vi "Associate Instruments to Paths.vi"(0 "SA Path Group in":refnum<class "SA Path Group.lvclass">, 5 "TSM Context":T1, 11 "error in":errorcluster) -> (4 "SA Path Group out":refnum<class "SA Path Group.lvclass">, 15 "error out":errorcluster)   [LabVIEW 2023, in "RFFixtureCharact.PXI.lvlib" / "SA Path Group.lvclass"]
uses:
  SA Path Group.lvclass
  SA Path Group.lvclass/SA Path Group.ctl
  Public/Base Classes/Scalar/SA Path/SA Path.lvclass
  <vilib>/NI_TestStand_SemiconductorModule/NI_TestStand_Semiconductor_Module.lvlibp
  Common/Base Classes/Path Group/Path Group.lvclass
  <vilib>/addons/_RFCalAndCharactDatabase/NI_RFCalAndCharact_Database_API.lvlibp/Characterization/Characterization.lvlib
  Common/RFCalAndFixtureCharact.Common.lvlib
  <vilib>/NI_TestStand_SemiconductorModule/NI_TestStand_Semiconductor_Module.lvlibp/PinMap/RF/RFmx/PinToNIRFmxSession.vi
  <vilib>/NI_TestStand_SemiconductorModule/NI_TestStand_Semiconductor_Module.lvlibp/PinMap/RF/RFSG/PinToNIRFSGSession.vi
  Public/Charact Result Accessor/Scalar/Scalar Charact Result Accessor.lvclass
  C:/rfcal/AuxTools/STSRFFixtureCharactUtility/Source/Code Modules/Fixture/Public/Charact Result Accessor/Base/Charact Result Accessor.lvclass
  C:/rfcal/AuxTools/STSRFFixtureCharactUtility/Source/Code Modules/Common/Result Accessor/Result Accessor.lvclass
  C:/rfcal/AuxTools/STSRFFixtureCharactUtility/Source/Code Modules/Fixture/Public/Charact Result Accessor/Scalar/Scalar Charact Result Accessor.lvclass
  C:/rfcal/AuxTools/STSRFFixtureCharactUtility/Source/Code Modules/Fixture/Public/Base Classes/Scalar/SA Abstract Path/SA Abstract Path.lvclass
  C:/rfcal/AuxTools/STSRFFixtureCharactUtility/Source/Code Modules/Fixture/Public/Base Classes/Scalar/Scalar Path/Scalar Path.lvclass
  C:/rfcal/AuxTools/STSRFFixtureCharactUtility/Source/Code Modules/Common/Base Classes/Path/Path.lvclass
  C:/rfcal/AuxTools/STSRFFixtureCharactUtility/Source/Code Modules/Fixture/Public/Base Classes/Scalar/SA Path/SA Path.lvclass
  <vilib>/NI_TestStand_SemiconductorModule/NI_TestStand_Semiconductor_Module.lvlibp/PinMap/General/SemiconductorModuleContext.ctl
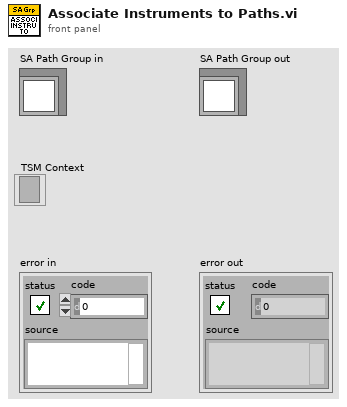
[diagram p1: front panel]
types:
  T1 = typedef "NI_TestStand_Semiconductor_Module.lvlibp/SemiconductorModuleContext.ctl" = refnum<k7>
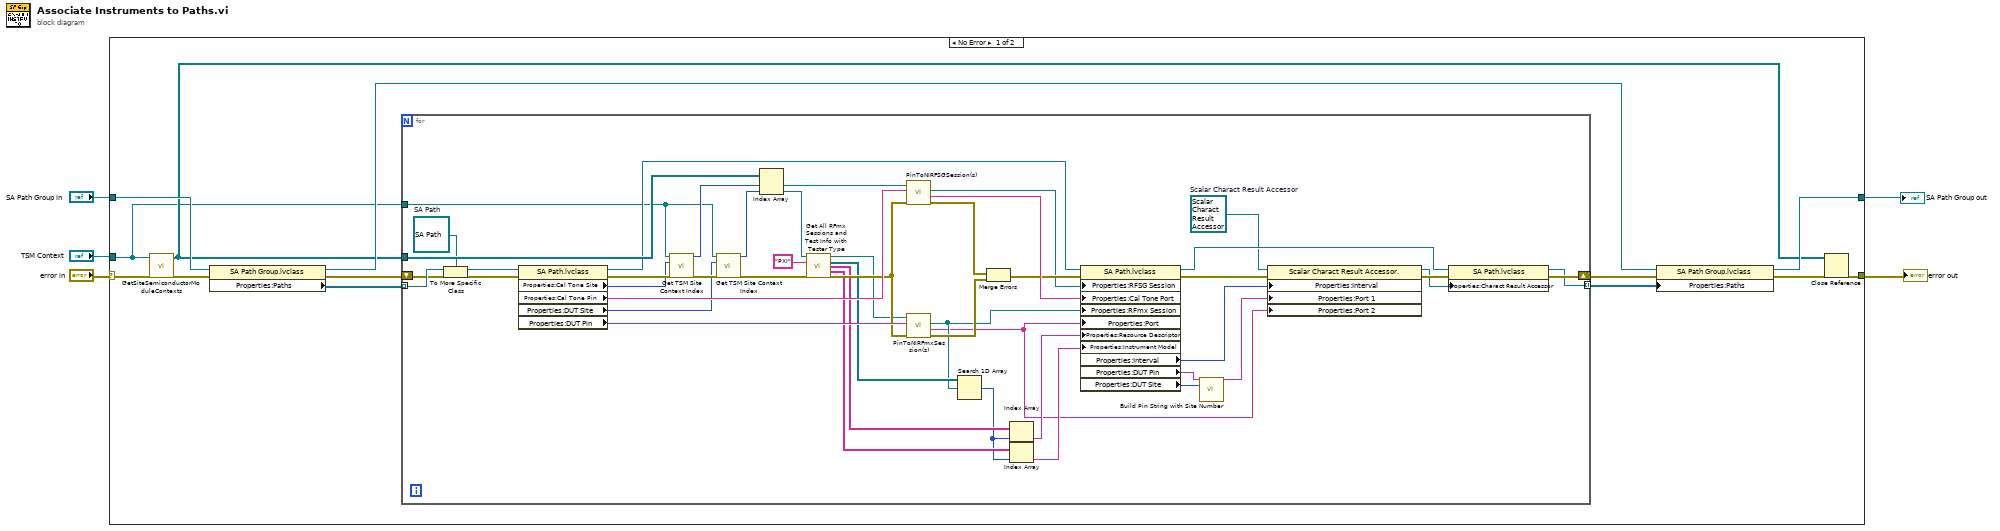
[diagram p0: block diagram]
diagram:
  n1 = case shown="No Error" "error in" {
    selector: "error in" -> [w10 w66]
    tunnel: "TSM Context" -> [w6 _]
    tunnel: "SA Path Group in" -> [w9 w65]
    tunnel: [w8 w66] -> w2
    tunnel: [w11 w65] -> w1
    frame No Error {
      n2 = call <vilib>:"GetSiteSemiconductorModuleContexts.vi"("error in (no error)"=w10, "Semiconductor Module Context"=w6) -> ("error out"=w15:errorcluster, "Site Semiconductor Module Contexts"=w7:T1[])  [unwired: 8 in]
      n3 = property class="SA Path Group.lvclass"(reference=w9, error in=w15) -> (reference out=w13:refnum<class "SA Path Group.lvclass">, error out=w17:errorcluster, "Properties:Paths"=w16:refnum<class "Path.lvclass">[])
      n4 = for {
        tunnel: w7 -> [w64]
        tunnel: w16 -> [w61] mode=indexing
        shift-right: [w51] -> w18
        shift-left: w17 -> [w57]
        tunnel: [w48] -> w12 mode=indexing
        tunnel: w6 -> [w41]
        w19 = refnum<class "Scalar Charact Result Accessor.lvclass"> refnum  # Scalar Charact Result Accessor
        w38 = refnum<class "SA Path.lvclass"> refnum  # SA Path
        n5 = To More Specific Class(target class=w38, reference=w61, error in=w57) -> (specific class reference=w58:refnum<class "SA Path.lvclass">, error out=w56:errorcluster)
        n6 = property class="SA Path.lvclass"(reference=w58, error in=w56) -> (reference out=w59:refnum<class "SA Path.lvclass">, error out=w55:errorcluster, "Properties:Cal Tone Site"=w42:i32, "Properties:Cal Tone Pin"=w43:string, "Properties:DUT Site"=w39:i32, "Properties:DUT Pin"=w40:string)
        n7 = call "Get TSM Site Context Index.vi"("Semiconductor Module Context"=w41, "Site Number"=w42, "error in (no error)"=w55) -> ("index of Site TSM Context"=w53:i32, "error out"=w46:errorcluster)  [unwired: 11 in]
        n8 = call "Get TSM Site Context Index.vi"("Semiconductor Module Context"=w41, "Site Number"=w39, "error in (no error)"=w46) -> ("index of Site TSM Context"=w45:i32, "error out"=w36:errorcluster)  [unwired: 11 in]
        n9 = Index Array(array=w64, index #1=w53, index #2=w45) -> (element #1=w44:T1, element #2=w33:T1)
        n10 = call "Get All RFmx Sessions and Test Info with Tester Type.vi"("TSM Context In"=w33, "Tester Type"="PXI", "error in"=w36) -> ("TSM Context Out"=w24:T1, "RFmx Sessions"=w32:refnum<k21>[], "Resource Descriptors"=w31:string[], "Instrument Models"=w29:string[], "error out"=w35:errorcluster)  [unwired: 8 in]
        n11 = call-poly <vilib>:"PinToNIRFSGSession(s).vi"("error in (no error)"=w35, "Pin"=w43, "Semiconductor Module Context"=w44) -> ("error out"=w60:errorcluster, "Port"=w63:string, "Instrument Session"=w37:refnum<k15>)  [unwired: 4 in, 2 out]
        n12 = call-poly <vilib>:"PinToNIRFmxSession(s).vi"("error in (no error)"=w35, "Pin"=w40, "Semiconductor Module Context"=w24) -> ("error out"=w54:errorcluster, "Port"=w25:string, "Instrument Session"=w26:refnum<k21>)  [unwired: 4 in, 2 out]
        n13 = Search 1D Array(1D array=w32, element=w26) -> (index of element=w27:i32)  [unwired: 1 in]
        n14 = Merge Errors(w60, w54) -> (w62:errorcluster)
        n15 = Index Array(array=w31, index=w27) -> (element=w30:string)
        n16 = Index Array(array=w29, index=w27) -> (element=w28:string)
        n17 = property class="SA Path.lvclass"(reference=w59, error in=w62, "Properties:RFSG Session"=w37, "Properties:Cal Tone Port"=w63, "Properties:RFmx Session"=w26, "Properties:Port"=w25, "Properties:Resource Descriptor"=w30, "Properties:Instrument Model"=w28) -> (reference out=w49:refnum<class "SA Path.lvclass">, error out=w20:errorcluster, "Properties:Interval"=w21:i32, "Properties:DUT Pin"=w23:string, "Properties:DUT Site"=w47:i32)
        n18 = call <vilib>:"Build Pin String with Site Number.vi"("Pin Name"=w23, "Site Number"=w47) -> ("Pin String"=w22:string)  [unwired: 13 in]
        n19 = property class="Scalar Charact Result Accessor."(reference=w19, error in=w20, "Properties:Interval"=w21, "Properties:Port 1"=w22, "Properties:Port 2"=w25) -> (reference out=w50:refnum<class "Scalar Charact Result Accessor.lvclass">, error out=w52:errorcluster)
        n20 = property class="SA Path.lvclass"(reference=w49, error in=w52, "Properties:Charact Result Accessor"=w50) -> (reference out=w48:refnum<class "SA Path.lvclass">, error out=w51:errorcluster)
      }
      n21 = property class="SA Path Group.lvclass"(reference=w13, error in=w18, "Properties:Paths"=w12) -> (reference out=w11:refnum<class "SA Path Group.lvclass">, error out=w14:errorcluster)
      n22 = Close Reference(reference=w7, error in (no error)=w14) -> (error out=w8:errorcluster)
    }
    frame Error {
    }
  }
  "error out" <- w2
  "SA Path Group out" <- w1
